vi "BRig_Host_dataRunState_entryAdd_DAB.vi"(7 "input_idx":i32[](array[numeric]), 9 "input_DAB_flipLR":u16, 10 "input_nTrial":u16, 11 "input_dataPlot":u16[][](array[numeric])) -> (3 "output_dataPlot":u16[][](array[numeric]), 5 "output_idx":i32[](array[numeric]))   [LabVIEW 2014]
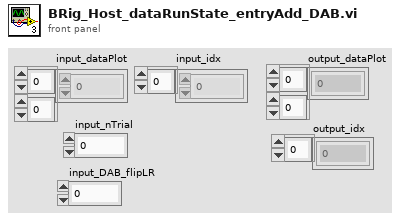
[diagram p1: front panel]
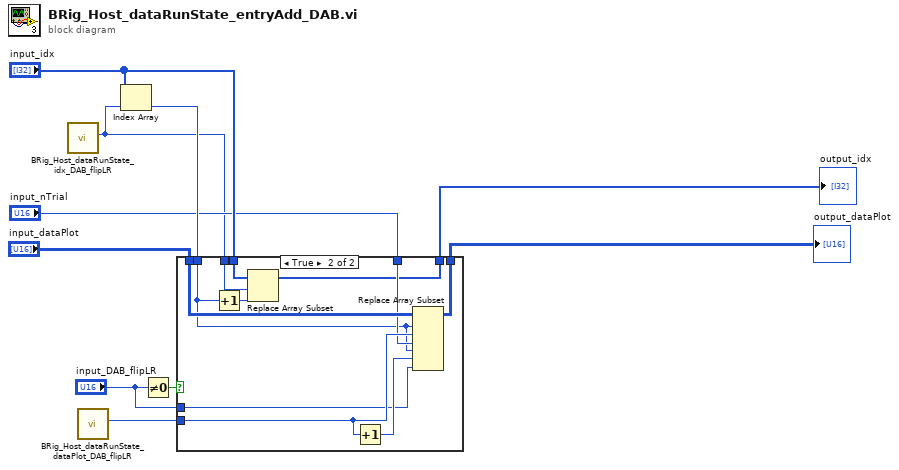
[diagram p0: block diagram]
diagram:
  n1 = call "BRig_Host_dataRunState_idx_DAB_flipLR.vi"() -> ("output_idx_DAB_flipLR"=w3:i32)  [unwired: 11 in]
  n2 = call "BRig_Host_dataRunState_dataPlot_DAB_flipLR.vi"() -> ("output_idx_dataPlot_DAB_flipLR"=w2:i32)  [unwired: 11 in]
  n3 = Index Array(array="input_idx", index=w3) -> (element=w8:i32)
  n4 = Not Equal To 0?(x="input_DAB_flipLR") -> (x != 0?=w10:bool)
  n5 = case shown="True" w10 {
    tunnel: w8 -> [_ w14]
    tunnel: "input_dataPlot" -> [w12 w23]
    tunnel: w2 -> [_ w22]
    tunnel: "input_nTrial" -> [_ w20]
    tunnel: [w12 w19] -> w4
    tunnel: w3 -> [_ w18]
    tunnel: "input_idx" -> [w11 w17]
    tunnel: [w11 w15] -> w5
    tunnel: "input_DAB_flipLR" -> [_ w13]
    frame False {
    }
    frame True {
      n6 = Increment(x=w14) -> (x+1=w16:i32)
      n7 = Replace Array Subset(array=w17, new element=w16, index=w18) -> (w15:i32[])
      n8 = Increment(x=w22) -> (x+1=w21:i32)
      n9 = Replace Array Subset(array=w23, new element #1=w20, index (row) #1=w14, index (col) #1=w22, new element #2=w13, index (row) #2=w14, index (col) #2=w21) -> (w19:u16[][])
    }
  }
  "output_dataPlot" <- w4
  "output_idx" <- w5
